vi "Test Positive Definite (CDB).vi"(10 "relative tolerance":dbl=-1.0, 11 "Input Matrix":T1) -> (0 "error":i32, 3 "positive definite?":bool)   [LabVIEW 2014, in "NI_AALPro.lvlib"]
uses:
  NI_AALPro.lvlib
  ComplexMatrix.ctl
  lvanlys.dll
  NI_Matrix.lvlib
panel:
  # "Test Positive Definite"
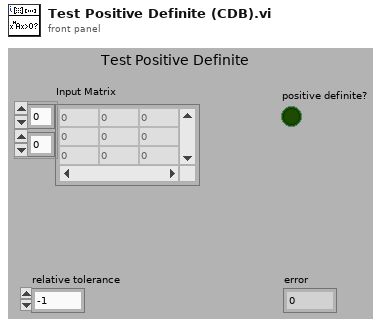
[diagram p1: front panel]
types:
  T1 = typedef "NI_Matrix.lvlib/ComplexMatrix.ctl" = cdb[][]
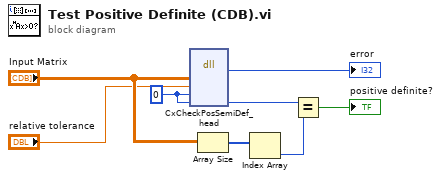
[diagram p0: block diagram]
diagram:
  w4 = 0 ("_possemidef")
  n1 = dll-call lib="C:/Program Files (x86)/National Instruments/LabVIEW 2014/resource/lvanlys.*" fn="CxCheckPosSemiDef_head"("_aH"="Input Matrix", "_tol"="relative tolerance", "_possemidef"=w4, "_rank"=w4) -> ("return type"=→"error":i32, "_rank"=w3:i32)  [unwired: 6 in, 2 out]
  n2 = Array Size(array="Input Matrix") -> (size(s)=w2:i32[])
  n3 = Index Array(array=w2) -> (element=w1:i32)  [unwired: 1 in]
  n4 = Equal?(x=w3, y=w1) -> (x = y?=→"positive definite?":bool)
